vi "Format Entry.vi"(8 "error in (no error)":errorcluster, 10 "Log Data":T1={"Time"=timestamp(0 s since 1904-01-01), "Level"=enum."INFO", "Logger"="", "Message"="", "Arguments"=[]} {"Time" format="%<%x %.3X>T"}, 11 "JSONLayout in":refnum<class "JSONLayout.lvclass">) -> (0 "error out":errorcluster, 2 "Log Entry":string, 3 "JSONLayout out":refnum<class "JSONLayout.lvclass">)   [LabVIEW 2019, in "TSC Event Logger.lvlib" / "JSONLayout.lvclass"]
uses:
  JSONLayout.lvclass
  Log Data.ctl
  Log/Event Level.ctl
  Layout.lvclass
  TSC Event Logger.lvlib
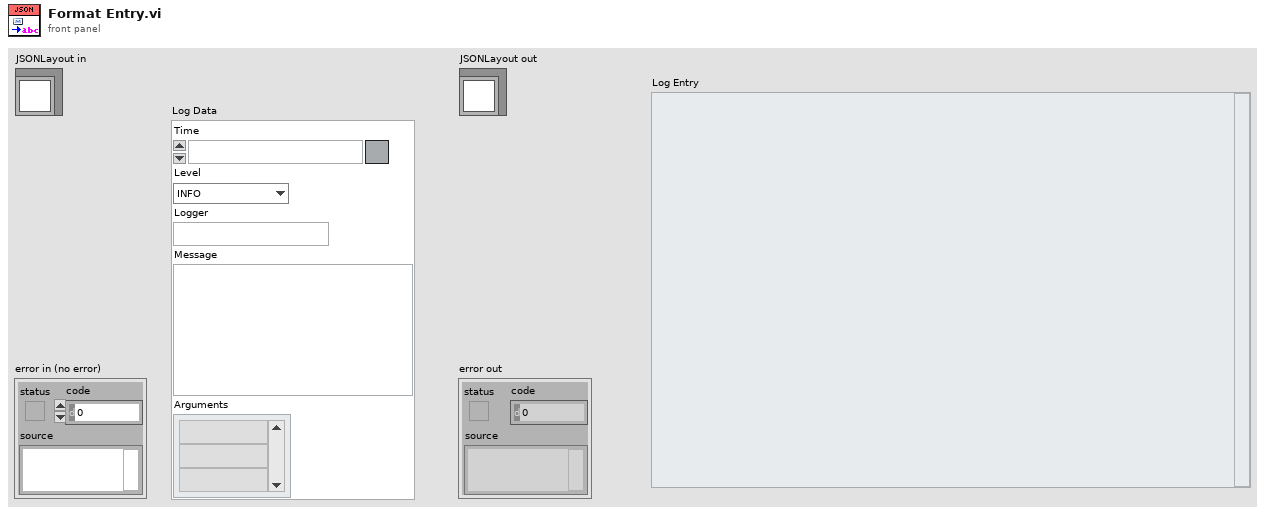
[diagram p1: front panel]
types:
  T1 = typedef "TSC Event Logger.lvlib/Log Data.ctl" = cluster{"Time":timestamp, "Level":T2, "Logger":string, "Message":string, "Arguments":string[]}
  T2 = typedef "TSC Event Logger.lvlib/Event Level.ctl" = enum16{"OFF", "TRACE", "DEBUG", "INFO", "WARN", "ERROR", "FATAL"}
  T3 = cluster{"Time":string, "Level":string, "Logger":string, "Message":string}
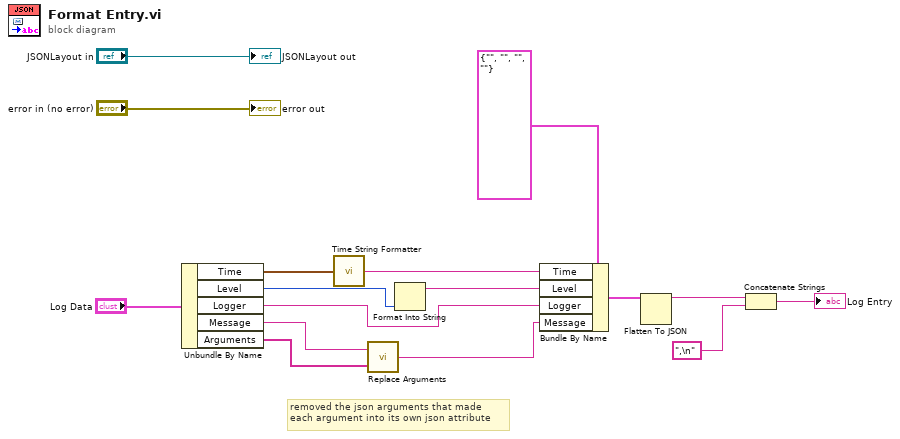
[diagram p0: block diagram]
diagram:
  # "removed the json arguments that made\neach argument into its own json attribute"
  n1 = Unbundle By Name("Log Data") -> ("Time"=w14:timestamp, "Level"=w8:T2, "Logger"=w6:string, "Message"=w13:string, "Arguments"=w12:string[])
  n2 = call "Time String Formatter.vi"("Time"=w14) -> ("Time string"=w9:string)
  n3 = call "Replace Arguments.vi"("Arguments"=w12, "Message"=w13) -> ("Output Message"=w3:string)
  n4 = Format Into String(w8) -> (resulting string=w7:string)  [unwired: 3 in, 1 out]
  n5 = Bundle By Name(cluster=T3 {"Time"="", "Level"="", "Logger"="", "Message"=""}, "Time"=w9, "Level"=w7, "Logger"=w6, "Message"=w3) -> (w5:T3)
  n6 = Flatten To JSON(anything=w5) -> (JSON string=w4:string)  [unwired: 2 in, 1 out]
  n7 = Concatenate Strings(w4, ",\n" ("string")) -> (→"Log Entry":string)
  "error out" <- "error in (no error)"
  "JSONLayout out" <- "JSONLayout in"
